vi "LVClass_Camera set all camera parameter values.vi"(0 "Camera in":refnum<class "Camera.lvclass">, 5 "CameraParametersSettable":T1[](array[typedef]), 7 "Image.lvclass new":refnum<class "Image.lvclass">, 11 "error in (no error)":errorcluster) -> (4 "Camera out":refnum<class "Camera.lvclass">, 15 "error out":errorcluster)   [LabVIEW 2020, in "Camera.lvclass"]
doc: "Set camera parameters which are settable parameter \n\n<B>CameraIn</B> : Camera object.\n<B>CameraOut</B> : Camera object.\n<B>BG Image OUIT</B> : image object to defined background image\n<B>ListOfSettableAndGettableValue</B> : Array of the parameter (name and value) to set to the camera."
uses:
  Camera.lvclass
  Image.lvclass
  CameraParametersSetup.ctl
  CameraParameters_Type.ctl
  Camera.lvclass/Camera.ctl
  LVClass_Camera Read acquisition state.vi
  LVClass_Camera Read all camera parameters.vi
  LVClass_Image read Image Compat ptr.vi
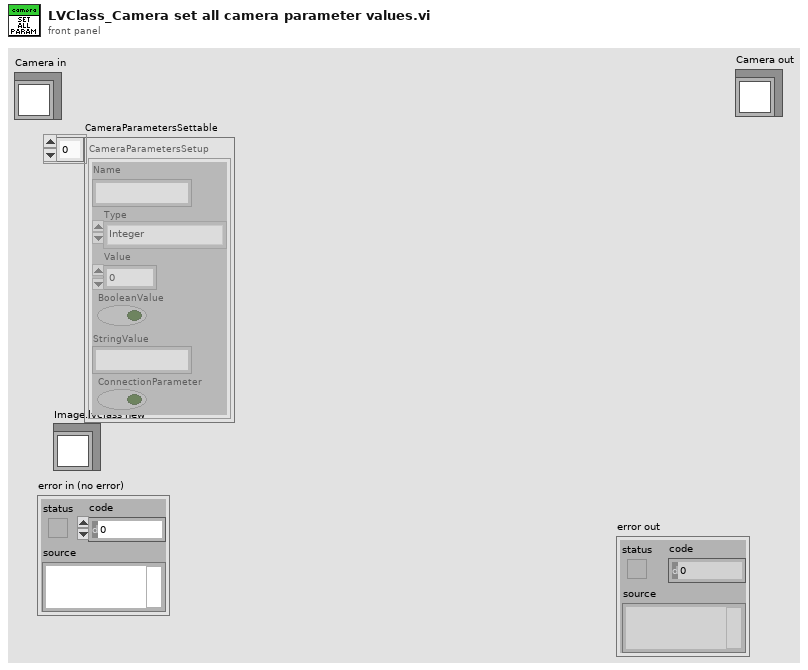
[diagram p1: front panel]
types:
  T1 = typedef "CameraParametersSetup.ctl" = cluster{"Name":string, "Type":T2, "Value":dbl, "BooleanValue":bool, "StringValue":string, "ConnectionParameter":bool}
  T2 = typedef "CameraParameters_Type.ctl" = enum16{"Integer", "Real", "String", "Boolean"}
  T3 = typedef "CameraAcquisitionState.ctl" = enum16{"Stop", "Live"}
  T4 = typedef "ParameterID.ctl" = cluster{"Name":string, "ConnectionParameter?":bool, "Type":T2, "Authorization":T5, "OnFlyAuthorization":T6, "StringValue":string, "Value":dbl, "Min":dbl, "Max":dbl, "BooleanValue":bool, "StringParameterList":string[]}
  T5 = typedef "CameraParameters_Authorization.ctl" = enum16{"Disable", "Gettable", "Settable - Gettable"}
  T6 = typedef "CameraParameters_OnFlyAuthorization.ctl" = enum16{"None", "Gettable", "Settable", "Settable - Gettable"}
  T7 = typedef "ClassID.ctl" = i64
  T8 = typedef "Image information.ctl" = cluster{"Image general information":T9, "Acquisition information":T10, "Number of pixels":T11, "Number of bits":T12}
  T9 = typedef "Image general information.ctl" = cluster{"Camera serial number":string, "Smearing removed":bool, "Background image removed":bool, "Time Stamp":timestamp, "Comment":string, "Camera_MAX_Level":i32}
  T10 = typedef "Image acquisition information.ctl" = cluster{"Exposure duration (us)":i32, "Exposure duration specified (us)":i32, "Gain":sgl, "Number of summed images":i32, "Trigger type":string}
  T11 = typedef "Point2D.ctl" = cluster{"X":u32, "Y":u32}
  T12 = typedef "Data alignment enum.ctl" = enum16{"8", "16", "32"}
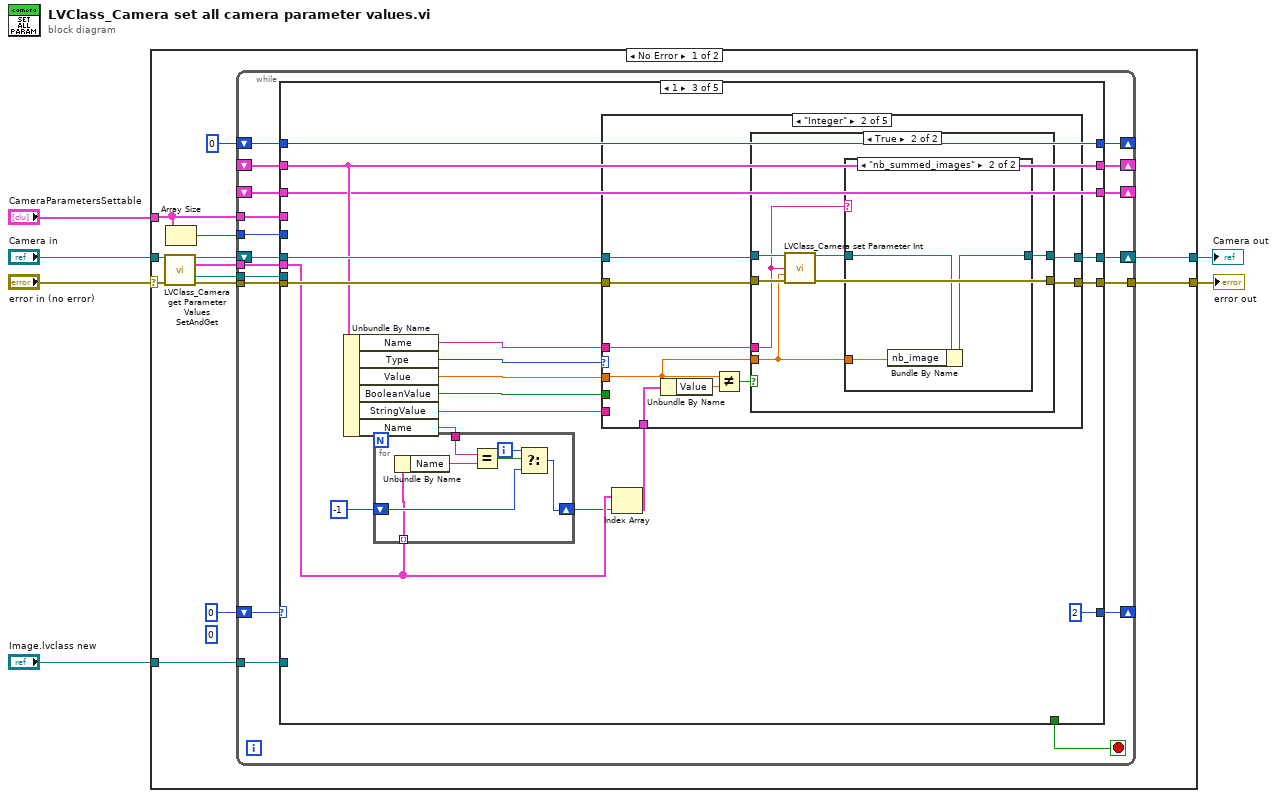
[diagram p0: block diagram]
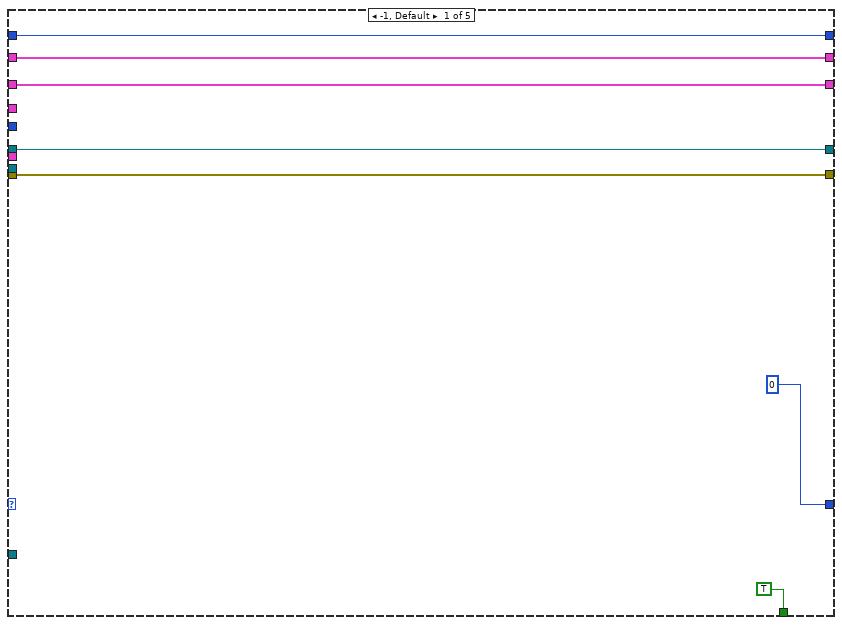
[diagram p2: hidden frame]
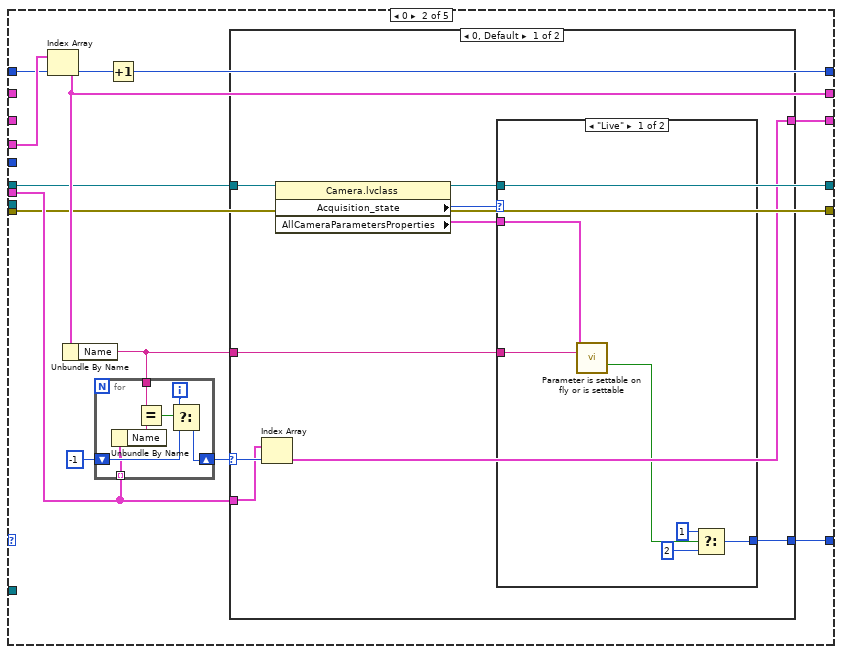
[diagram p3: hidden frame]
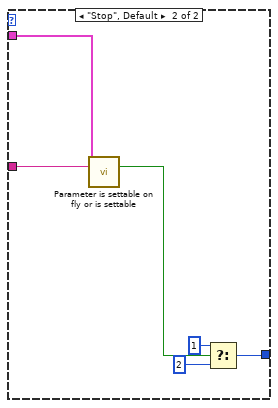
[diagram p4: hidden frame]
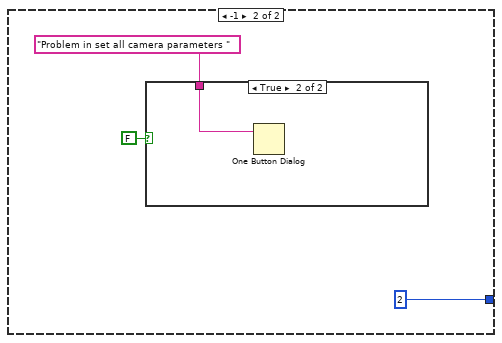
[diagram p5: hidden frame]
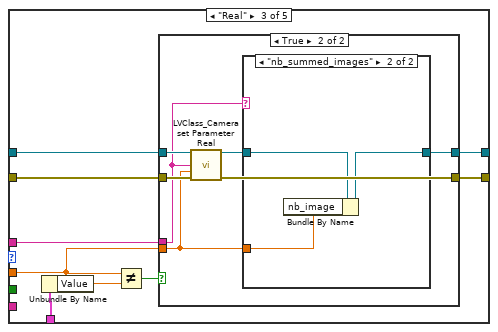
[diagram p10: hidden frame]
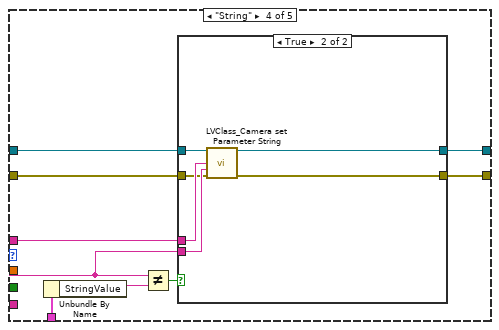
[diagram p13: hidden frame]
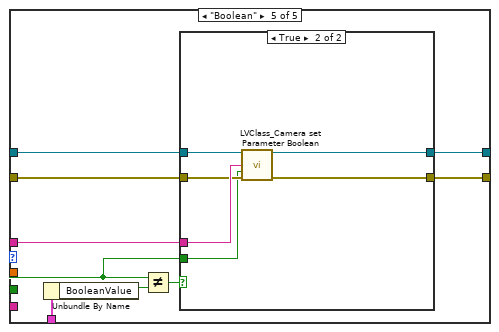
[diagram p15: hidden frame]
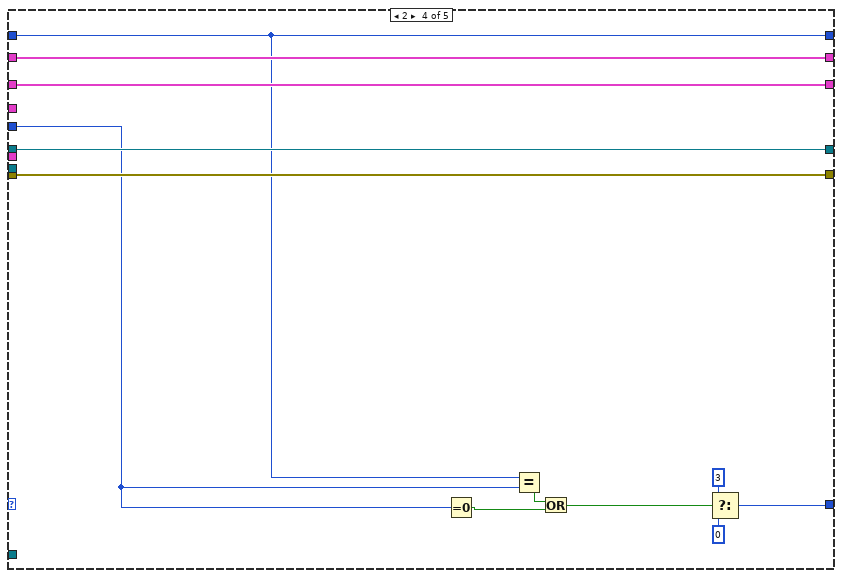
[diagram p17: hidden frame]
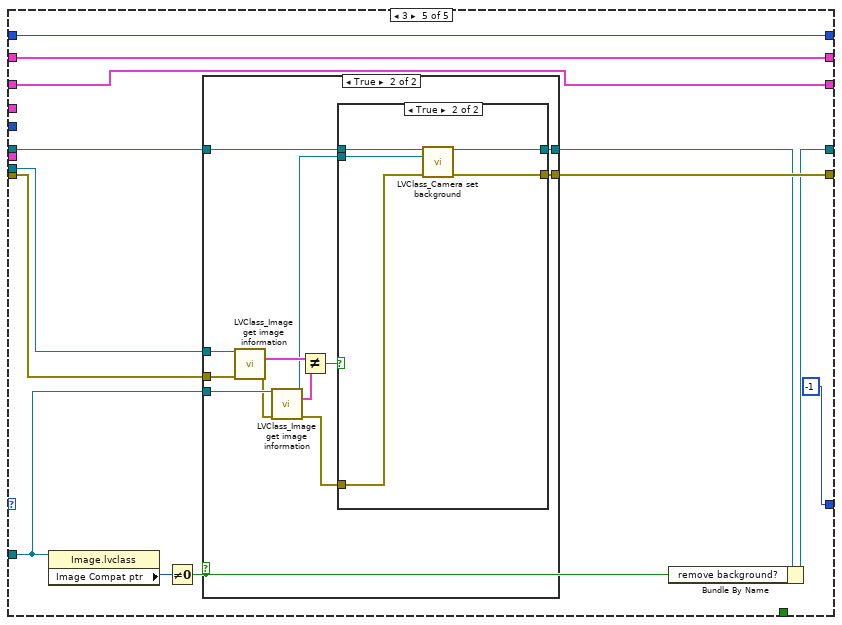
[diagram p18: hidden frame]
diagram:
  n1 = case shown="No Error" "error in (no error)" {
    selector: "error in (no error)" -> [w19 w241]
    tunnel: [w12 w241] -> w5
    tunnel: [w14 w240] -> w4
    tunnel: "Camera in" -> [w18 w240]
    tunnel: "CameraParametersSettable" -> [w8 _]
    tunnel: "Image.lvclass new" -> [w10 _]
    frame No Error {
      (unwired) 0
      n2 = call "LVClass_Camera get Parameter Values SetAndGet.vi"("Camera in"=w18, "error in (no error)"=w19) -> ("Camera out"=w15:refnum<class "Camera.lvclass">, "ListOfSettableAndGettableValue"=w13:T1[], "BG Image OUT"=w11:refnum<class "Image.lvclass">, "error out"=w17:errorcluster)  [unwired: 10 in]
      n3 = Array Size(array=w8) -> (size(s)=w7:i32)
      n4 = while {
        tunnel: w17 -> [w33]
        shift-right: [w36] -> _
        shift-left: 0 -> [w37]
        tunnel: w13 -> [w31]
        tunnel: [w32] -> w12
        tunnel: w8 -> [w30]
        tunnel: w11 -> [w29]
        tunnel: w10 -> [w28]
        shift-right: [w34] -> w14
        shift-left: w15 -> [w35]
        shift-right: [w23] -> _
        shift-left: 0 -> [w26]
        shift-right: [w25] -> _
        shift-left: _ -> [w24]
        tunnel: w7 -> [w22]
        shift-right: [w21] -> _
        shift-left: _ -> [w20]
        stop <- w27 stop-if-true
        n5 = case shown="1" w37 {
          tunnel: [0 w49 2 w200 -1] -> w36
          tunnel: w35 -> [w44 w48 w105 w203 w217]
          tunnel: [w44 w48 w104 w203 w214] -> w34
          tunnel: w33 -> [w43 w51 w103 w202 w211]
          tunnel: [w43 w51 w102 w202 w216] -> w32
          tunnel: w31 -> [_ w56 w101 _ _]
          tunnel: w30 -> [_ w53 _ _ _]
          tunnel: w29 -> [_ _ _ _ w213]
          tunnel: w28 -> [_ _ _ _ w212]
          tunnel: [TRUE _ _ _ _] -> w27
          tunnel: w26 -> [w38 w50 w91 w201 w206]
          tunnel: [w40 w52 w100 w205 w208] -> w25
          tunnel: w24 -> [w40 _ w100 w205 w208]
          tunnel: [w38 w46 w91 w201 w206] -> w23
          tunnel: w22 -> [_ _ _ w197 _]
          tunnel: [w39 w45 w89 w204 w207] -> w21
          tunnel: w20 -> [w39 _ w89 w204 w207]
          frame -1, Default {
          }
          frame 0 {
            n6 = Index Array(array=w53, index=w50) -> (element=w52:T1)
            n7 = Unbundle By Name(w52) -> ("Name"=w47:string)
            n8 = for {
              tunnel: w47 -> [w87]
              shift-right: [w84] -> w54
              shift-left: -1 -> [w83]
              tunnel: w56 -> [w82] mode=indexing
              i -> [w85]
              n9 = Unbundle By Name(w82) -> ("Name"=w88:string)
              n10 = Equal?(x=w87, y=w88) -> (x = y?=w86:bool)
              n11 = Select(t=w85, s=w86, f=w83) -> (s? t:f=w84:i32)
            }
            n12 = Increment(x=w50) -> (x+1=w46:i32)
            n13 = case shown="0, Default" w54 {
              selector: w54 -> [w63 _]
              tunnel: w56 -> [w62 _]
              tunnel: [w65 2] -> w49
              tunnel: w48 -> [w64 _]
              tunnel: w47 -> [w59 _]
              tunnel: [w61 _] -> w45
              frame 0, Default {
                n14 = Index Array(array=w62, index=w63) -> (element=w61:T1)
                n15 = property class="Camera.lvclass"(reference=w64) -> (reference out=w58:refnum<class "Camera.lvclass">, "Acquisition_state"=w60:T3, "AllCameraParametersProperties"=w57:T4[])  [unwired: 1 in, 1 out]
                n16 = case shown="\"Live\"" w60 {
                  tunnel: [w70 w76] -> w65
                  tunnel: w59 -> [w71 w77]
                  tunnel: w58 -> [_ _]
                  tunnel: w57 -> [w66 w73]
                  frame "Live" {
                    n17 = call "Parameter is settable on fly or is settable.vi"("AllCameraParameters"=w66, "Name"=w71) -> ("SettableOnLive?"=w67:bool)  [unwired: 11 in, 2 out]
                    n18 = Select(t=1, s=w67, f=2) -> (s? t:f=w70:i32)
                  }
                  frame "Stop", Default {
                    n19 = call "Parameter is settable on fly or is settable.vi"("AllCameraParameters"=w73, "Name"=w77) -> ("Settable?"=w72:bool)  [unwired: 11 in, 2 out]
                    n20 = Select(t=1, s=w72, f=2) -> (s? t:f=w76:i32)
                  }
                }
              }
              frame -1 {
                n21 = case shown="True" FALSE {
                  tunnel: "Problem in set all camera parameters " ("message") -> [_ w81]
                  frame False {
                  }
                  frame True {
                    n22 = One Button Dialog(message=w81) -> ()  [unwired: 1 in, 1 out]
                  }
                }
              }
            }
          }
          frame 1 {
            n23 = Unbundle By Name(w100) -> ("Name"=w94:string, "Type"=w99:T2, "Value"=w95:dbl, "BooleanValue"=w97:bool, "StringValue"=w96:string, "Name"=w93:string)
            n24 = for {
              tunnel: w93 -> [w192]
              shift-right: [w189] -> w92
              shift-left: -1 -> [w188]
              tunnel: w101 -> [w187] mode=indexing
              i -> [w190]
              n25 = Unbundle By Name(w187) -> ("Name"=w193:string)
              n26 = Equal?(x=w192, y=w193) -> (x = y?=w191:bool)
              n27 = Select(t=w190, s=w191, f=w188) -> (s? t:f=w189:i32)
            }
            n28 = Index Array(array=w101, index=w92) -> (element=w90:T1)
            n29 = case shown="\"Integer\"" w99 {
              tunnel: w94 -> [_ w110 w132 w159 w176]
              tunnel: w105 -> [w108 w116 w138 w160 w177]
              tunnel: [w108 w114 w136 w157 w174] -> w104
              tunnel: [w107 w113 w135 w156 w173] -> w102
              tunnel: w103 -> [w107 w115 w137 w158 w175]
              tunnel: w90 -> [_ w117 w139 w161 w178]
              tunnel: w95 -> [_ w112 w133 _ _]
              tunnel: w97 -> [_ _ _ _ w170]
              tunnel: w96 -> [_ _ _ w153 _]
              frame Default {
              }
              frame "Integer" {
                n30 = Unbundle By Name(w117) -> ("Value"=w111:dbl)
                n31 = Not Equal?(x=w112, y=w111) -> (x != y?=w109:bool)
                n32 = case shown="True" w109 {
                  tunnel: w116 -> [w119 w126]
                  tunnel: w110 -> [_ w123]
                  tunnel: w115 -> [w118 w125]
                  tunnel: [w119 w122] -> w114
                  tunnel: [w118 w124] -> w113
                  tunnel: w112 -> [_ w120]
                  frame False {
                  }
                  frame True {
                    n33 = call "LVClass_Camera set Parameter Int.vi"("Camera in"=w126, "parameter_name"=w123, "value"=w120, "error in (no error)"=w125) -> ("Camera out"=w121:refnum<class "Camera.lvclass">, "error out"=w124:errorcluster)  [unwired: 10 in]
                    n34 = case shown="\"nb_summed_images\"" w123 {
                      tunnel: [w127 w129] -> w122
                      tunnel: w121 -> [w127 w130]
                      tunnel: w120 -> [_ w128]
                      frame Default {
                      }
                      frame "nb_summed_images" {
                        n35 = Bundle By Name(cluster=w130, "nb_image"=w128) -> (w129:refnum<class "Camera.lvclass">)
                      }
                    }
                  }
                }
              }
              frame "Real" {
                n36 = Unbundle By Name(w139) -> ("Value"=w134:dbl)
                n37 = Not Equal?(x=w133, y=w134) -> (x != y?=w131:bool)
                n38 = case shown="True" w131 {
                  tunnel: w138 -> [w141 w148]
                  tunnel: w132 -> [_ w142]
                  tunnel: w137 -> [w140 w147]
                  tunnel: [w141 w145] -> w136
                  tunnel: [w140 w144] -> w135
                  tunnel: w133 -> [_ w143]
                  frame False {
                  }
                  frame True {
                    n39 = call "LVClass_Camera set Parameter Real.vi"("Camera in"=w148, "parameter_name"=w142, "value"=w143, "error in (no error)"=w147) -> ("Camera out"=w146:refnum<class "Camera.lvclass">, "error out"=w144:errorcluster)  [unwired: 10 in]
                    n40 = case shown="\"nb_summed_images\"" w142 {
                      tunnel: [w149 w151] -> w145
                      tunnel: w146 -> [w149 w152]
                      tunnel: w143 -> [_ w150]
                      frame Default {
                      }
                      frame "nb_summed_images" {
                        n41 = Bundle By Name(cluster=w152, "nb_image"=w150) -> (w151:refnum<class "Camera.lvclass">)
                      }
                    }
                  }
                }
              }
              frame "String" {
                n42 = Unbundle By Name(w161) -> ("StringValue"=w154:string)
                n43 = Not Equal?(x=w153, y=w154) -> (x != y?=w155:bool)
                n44 = case shown="True" w155 {
                  tunnel: w160 -> [w163 w169]
                  tunnel: w159 -> [_ w166]
                  tunnel: w158 -> [w162 w164]
                  tunnel: [w163 w168] -> w157
                  tunnel: [w162 w167] -> w156
                  tunnel: w153 -> [_ w165]
                  frame False {
                  }
                  frame True {
                    n45 = call "LVClass_Camera set Parameter String.vi"("Camera in"=w169, "parameter_name"=w166, "value"=w165, "error in (no error)"=w164) -> ("Camera out"=w168:refnum<class "Camera.lvclass">, "error out"=w167:errorcluster)  [unwired: 10 in]
                  }
                }
              }
              frame "Boolean" {
                n46 = Unbundle By Name(w178) -> ("BooleanValue"=w171:bool)
                n47 = Not Equal?(x=w170, y=w171) -> (x != y?=w172:bool)
                n48 = case shown="True" w172 {
                  tunnel: w177 -> [w180 w186]
                  tunnel: w176 -> [_ w184]
                  tunnel: w175 -> [w179 w183]
                  tunnel: [w180 w185] -> w174
                  tunnel: [w179 w182] -> w173
                  tunnel: w170 -> [_ w181]
                  frame False {
                  }
                  frame True {
                    n49 = call "LVClass_Camera set Parameter Boolean.vi"("Camera in"=w186, "parameter_name"=w184, "value"=w181, "error in (no error)"=w183) -> ("Camera out"=w185:refnum<class "Camera.lvclass">, "error out"=w182:errorcluster)  [unwired: 10 in]
                  }
                }
              }
            }
          }
          frame 2 {
            n50 = Equal To 0?(x=w197) -> (x = 0?=w196:bool)
            n51 = Equal?(x=w201, y=w197) -> (x = y?=w195:bool)
            n52 = Or(x=w195, y=w196) -> (x .or. y?=w194:bool)
            n53 = Select(t=3, s=w194, f=0) -> (s? t:f=w200:i32)
          }
          frame 3 {
            n54 = property class="Image.lvclass"(reference=w212) -> ("Image Compat ptr"=w210:T7)  [unwired: 1 in, 2 out]
            n55 = Not Equal To 0?(x=w210) -> (x != 0?=w209:bool)
            n56 = case shown="True" w209 {
              tunnel: w217 -> [w220 w231]
              tunnel: [w219 w230] -> w216
              tunnel: [w220 w229] -> w215
              tunnel: w213 -> [_ w228]
              tunnel: w212 -> [_ w227]
              tunnel: w211 -> [w219 w225]
              frame False {
              }
              frame True {
                n57 = call "LVClass_Image get image information.vi"("Image in"=w228, "error in (no error)"=w225) -> ("Acquisition information"=w223:T8, "error out"=w226:errorcluster)  [unwired: 11 in, 1 out]
                n58 = call "LVClass_Image get image information.vi"("Image in"=w227, "error in (no error)"=w226) -> ("Image out"=w221:refnum<class "Image.lvclass">, "Acquisition information"=w222:T8, "error out"=w224:errorcluster)  [unwired: 11 in]
                n59 = Not Equal?(x=w223, y=w222) -> (x != y?=w232:bool)
                n60 = case shown="True" w232 {
                  tunnel: w231 -> [w234 w239]
                  tunnel: w224 -> [w233 w237]
                  tunnel: w221 -> [_ w238]
                  tunnel: [w234 w236] -> w229
                  tunnel: [w233 w235] -> w230
                  frame False {
                  }
                  frame True {
                    n61 = call "LVClass_Camera set background.vi"("Camera in"=w239, "Image.lvclass"=w238, "error in (no error)"=w237) -> ("Camera out"=w236:refnum<class "Camera.lvclass">, "error out"=w235:errorcluster)  [unwired: 11 in]
                  }
                }
              }
            }
            n62 = Bundle By Name(cluster=w215, "remove background?"=w209) -> (w214:refnum<class "Camera.lvclass">)
          }
        }
      }
    }
    frame Error {
    }
  }
  "error out" <- w5
  "Camera out" <- w4
